vi "Variant Global.vi"() -> ()   [LabVIEW 2013, in "TS.lvlib"]
uses:
  TS.lvlib
panel:
  out "Attribute Storage":variant
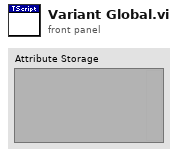
[diagram p1: front panel]
diagram:
